vi "Funct TIFF export-Bring to front.vi"   [LabVIEW 2017]
uses:
  Globals/gl_funct TIFF export globals.vi
types:
  T1 = typedef "Funct TIFF exporter ctrl refs.ctl" = cluster{"This VI":refnum<vi>, "Current Experiment":refnum<vi>, "Imaging protocol":refnum<vi>, "Predominant ROI type":refnum<vi>, "Patches in Experiment":refnum<vi>, "Folder Path":refnum<vi>, "Export":refnum<vi>, "Trial number":refnum<vi>, "Output TIFF type":refnum<vi>}
  T2 = enum32{"Invalid", "Standard", "Closed", "Hidden", "Minimized", "Maximized"}
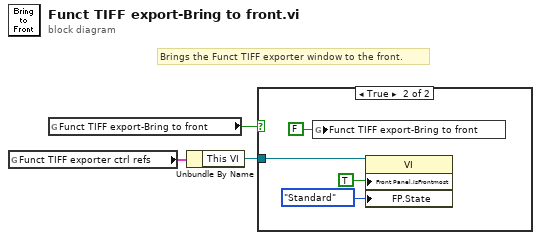
[diagram p0: block diagram]
diagram:
  # "Brings the Funct TIFF exporter window to the front."
  n1 = global read "gl_funct TIFF export globals.vi" "Funct TIFF exporter ctrl refs"() -> (w1:T1)
  n2 = global read "gl_funct TIFF export globals.vi" "Funct TIFF export-Bring to front"() -> (w2:bool)
  n3 = Unbundle By Name(w1) -> ("This VI"=w3:refnum<vi>)
  n4 = case shown="True" w2 {
    tunnel: w3 -> [_ w5]
    frame False {
    }
    frame True {
      n5 = global write "gl_funct TIFF export globals.vi" "Funct TIFF export-Bring to front"(FALSE ("Funct TIFF export-Bring to front")) -> ()
      n6 = property class="VI"(reference=w5, "Front Panel.IsFrontmost"=TRUE ("Front Panel Window:Is Frontmost"), "FP.State"=T2."Standard" ("Front Panel Window:State")) -> ()  [unwired: 1 in, 2 out]
    }
  }
